vi "Do.vi"(8 "error in (no error)":errorcluster, 10 "DataExchange":T1, 11 "QuickNote in":refnum<class "QuickNote.lvclass">) -> (0 "error out":errorcluster, 2 "DataExchange Out":T1, 3 "QuickNote out":refnum<class "QuickNote.lvclass">)   [LabVIEW 2020, in "QuickNote.lvlib" / "QuickNote.lvclass"]
uses:
  QuickNote.lvclass
  <vilib>/vision/Image Controls.llb/IMAQ Image.ctl
  Hardware Abstraction Layer/Component/GRMActor/GRMActor/GRMActor.lvclass
  Hardware Abstraction Layer/Component/Device/Device/DataExchange.ctl
  Interface/DataListener/DataListener.lvclass
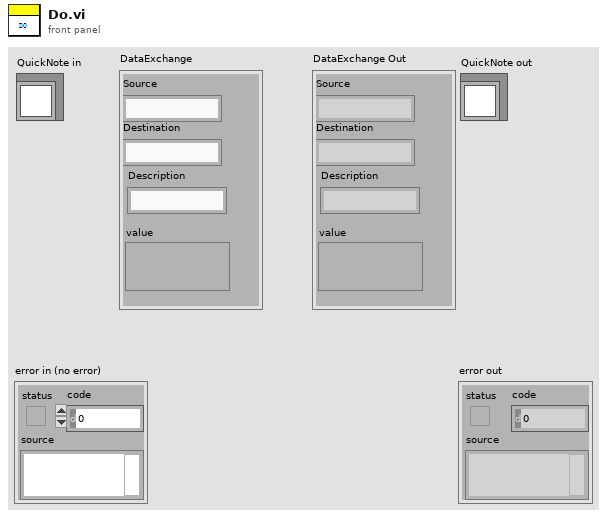
[diagram p1: front panel]
types:
  T1 = typedef "DataListener.lvclass/DataExchange.ctl" = cluster{"Source":string, "Destination":string, "Description":string, "value":variant}
  T2 = typedef "IMAQ Image.ctl" = refnum<image>
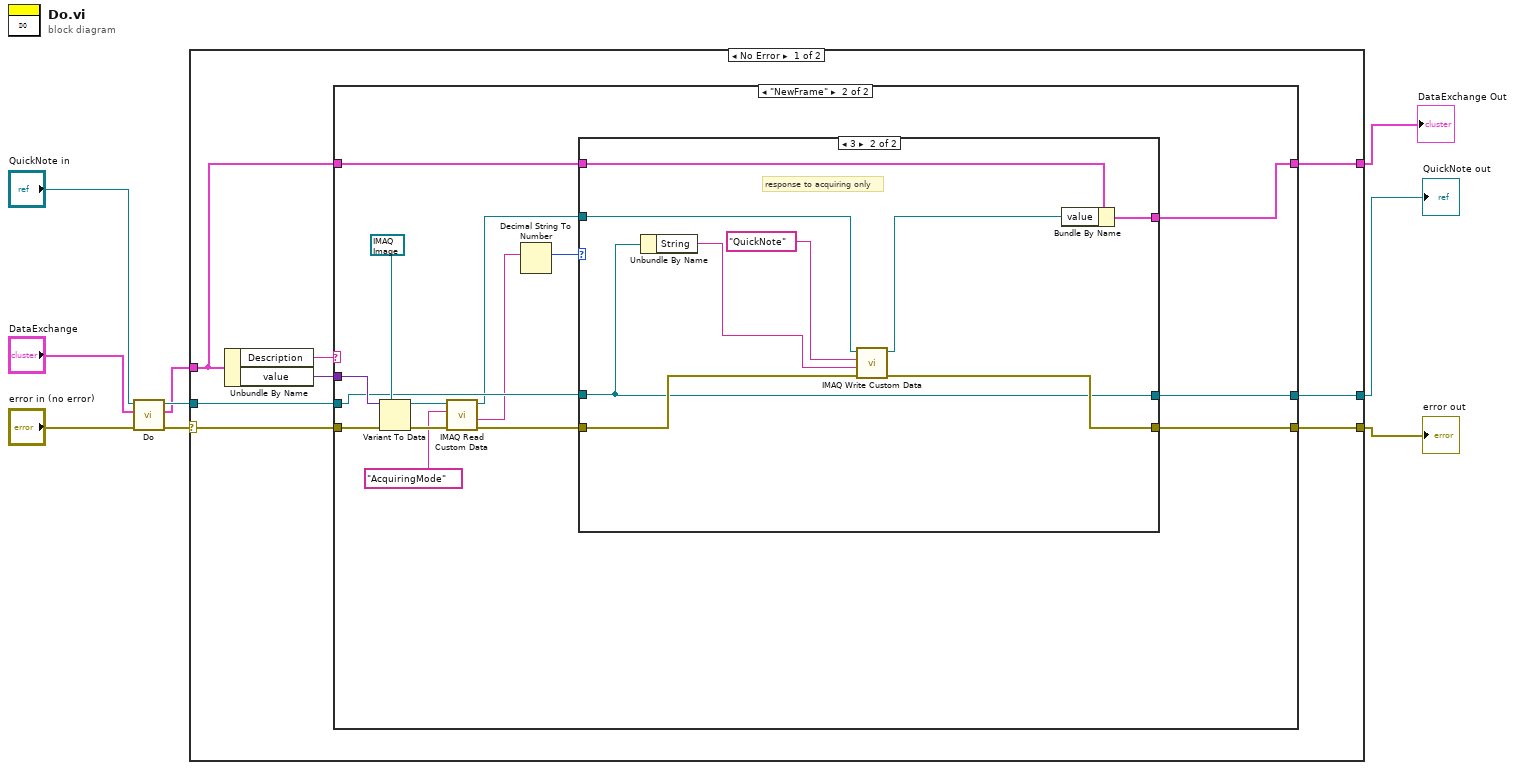
[diagram p0: block diagram]
diagram:
  n1 = call-parent "Do.vi"("error in (no error)"="error in (no error)", "DataExchange"="DataExchange", "DataProcessor in"="QuickNote in") -> ("error out"=w6:errorcluster, "DataExchange Out"=w4:T1, "DataProcessor out"=w5:refnum<class "QuickNote.lvclass">)  [unwired: 6 in]
  n2 = case shown="No Error" w6 {
    selector: w6 -> [w15 w50]
    tunnel: [w16 w50] -> w3
    tunnel: w5 -> [w12 w49]
    tunnel: [w17 w49] -> w2
    tunnel: w4 -> [w11 w48]
    tunnel: [w10 w48] -> w1
    frame No Error {
      n3 = Unbundle By Name(w11) -> ("Description"=w14:string, "value"=w13:variant)
      n4 = case shown="\"NewFrame\"" w14 {
        tunnel: w13 -> [_ w34]
        tunnel: [w20 w24] -> w17
        tunnel: w12 -> [w20 w25]
        tunnel: [w19 w26] -> w16
        tunnel: w15 -> [w19 w35]
        tunnel: w11 -> [w18 w31]
        tunnel: [w18 w30] -> w10
        frame Default {
        }
        frame "NewFrame" {
          n5 = Variant To Data(error in=w35, type=T2 refnum ("New Image"), Variant=w34) -> (data=w28:T2, error out=w32:errorcluster)
          n6 = call "IMAQ Read Custom Data"("error in (no error)"=w32, "Key"="AcquiringMode", "Image"=w28) -> ("error out"=w29:errorcluster, "Custom Data Out"=w22:string, "Image (duplicate)"=w23:T2)  [unwired: 6 in]
          n7 = Decimal String To Number(string=w22) -> (number=w21:i32)  [unwired: 2 in, 1 out]
          n8 = case shown="3" w21 {
            tunnel: w31 -> [w38 w47]
            tunnel: [w38 w46] -> w30
            tunnel: w29 -> [w36 w45]
            tunnel: w23 -> [_ w43]
            tunnel: [w36 w44] -> w26
            tunnel: w25 -> [w37 w42]
            tunnel: [w37 w42] -> w24
            frame Default {
            }
            frame 3 {
              # "response to acquiring only"
              n9 = Unbundle By Name(w42) -> ("String"=w39:string)
              n10 = call "IMAQ Write Custom Data"("error in (no error)"=w45, "Custom Data In"=w39, "Key"="QuickNote", "Image"=w43) -> ("error out"=w44:errorcluster, "Image Out"=w40:T2)  [unwired: 6 in]
              n11 = Bundle By Name(cluster=w47, "value"=w40) -> (w46:T1)
            }
          }
        }
      }
    }
    frame Error {
    }
  }
  "error out" <- w3
  "QuickNote out" <- w2
  "DataExchange Out" <- w1
